vi "Parse SVM Timer Args.vi"(7 "Flame?":bool, 9 "State String":string) -> (1 "Timer Inputs":T1, 2 "State String out":string)   [LabVIEW 2013]
doc: "This sub-VI parses an input state string of the form \"state:target:relight\" and outputs a timer_input_cluster\nobject comprising the arguments \"target\", which is a float indicating a target time, and \"relight\" which is a\nBoolean. Note that \"relight\" must be \"T\" to return a True value, and anything else (\"F\" preferred) for False."
uses:
  Controls/timer_input_cluster.ctl
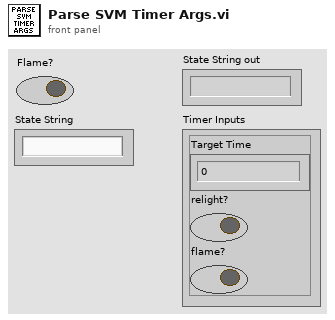
[diagram p1: front panel]
types:
  T1 = typedef "timer_input_cluster.ctl" = cluster{"Target Time":dbl, "relight?":bool, "flame?":bool}
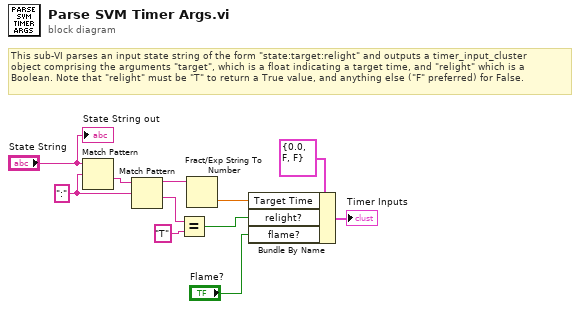
[diagram p0: block diagram]
diagram:
  w9 = ":" ("regular expression")
  # "This sub-VI parses an input state string of the form \"state:target:relight\" and outputs a timer_input_cluster\nobject comprising the arguments \"target\", which is a float indicating a target time, and \"relight\" which is a\nBoolean. Note that \"relight\" must be \"T\" to return a True value, and anything else (\"F\" preferred) for False."
  n1 = Match Pattern(string="State String", regular expression=w9) -> (after substring=w10:string)  [unwired: 1 in, 3 out]
  n2 = Match Pattern(string=w10, regular expression=w9) -> (before substring=w8:string, after substring=w6:string)  [unwired: 1 in, 2 out]
  n3 = Equal?(x=w6, y="T") -> (x = y?=w4:bool)
  n4 = Fract/Exp String To Number(string=w8) -> (number=w7:dbl)  [unwired: 3 in, 1 out]
  n5 = Bundle By Name(cluster=T1 {"Target Time"=0.0, "relight?"=FALSE, "flame?"=FALSE} ("Timer Inputs 2"), "Target Time"=w7, "relight?"=w4, "flame?"="Flame?") -> (→"Timer Inputs":T1)
  "State String out" <- "State String"
